vi "CRYNL Interpolation.vi"(10 "y in":dbl[](array[numeric]), 11 "x in":dbl[](array[numeric])) -> (2 "y out":dbl[](array[numeric]))   [LabVIEW 2013]
uses:
  <vilib>/Analysis/4window.llb/Hanning Window (DBL).vi
  <vilib>/Analysis/4window.llb/AllCosWindow (DBL).vi
  <vilib>/Analysis/NI_AALPro.lvlib
panel:
  out "Raw and Interpolated Data":cluster{"x in":dbl[], "y in":dbl[]}[](graph)
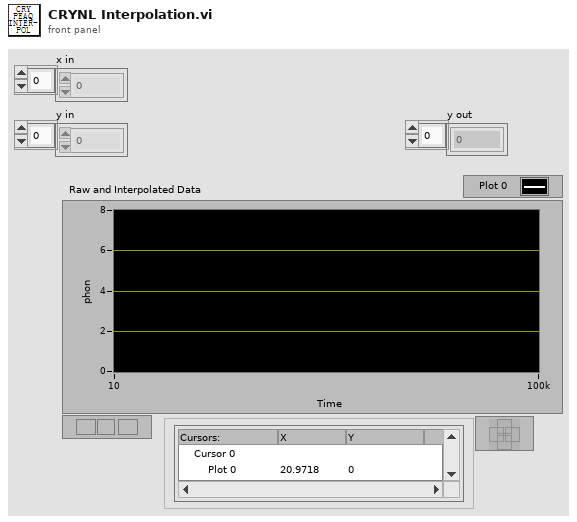
[diagram p1: front panel]
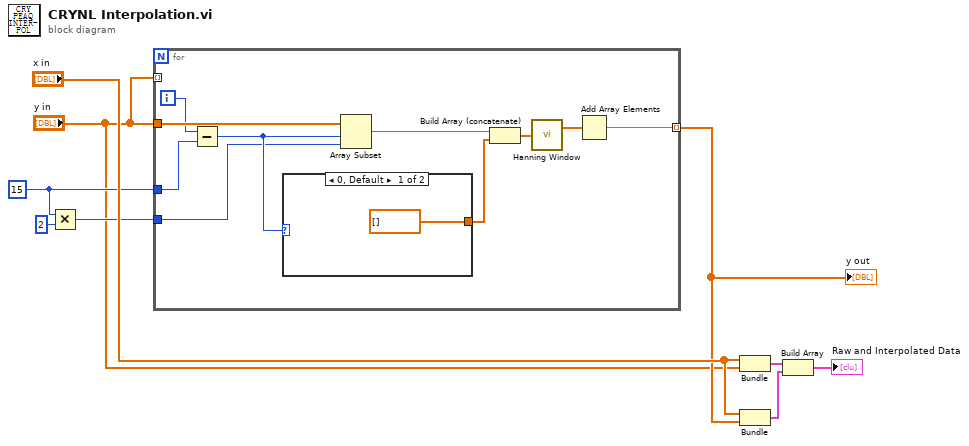
[diagram p0: block diagram]
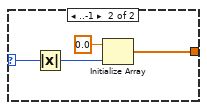
[diagram p2: hidden frame]
diagram:
  w6 = 15 ("y")
  n1 = Multiply(x=w6, y=2) -> (x*y=w4:i32)
  n2 = for {
    tunnel: "y in" -> [w19]
    tunnel: w6 -> [w17]
    tunnel: [w16] -> w3 mode=indexing
    tunnel: w4 -> [w14]
    tunnel: "y in" -> [_] mode=indexing
    i -> [w18]
    n3 = Subtract(x=w18, y=w17) -> (x-y=w15:i32)
    n4 = case shown="0, Default" w15 {
      selector: w15 -> [_ w24]
      tunnel: [dbl[] [] w21] -> w12
      frame 0, Default {
      }
      frame ..-1 {
        n5 = Absolute Value(x=w24) -> (abs(x)=w22:i32)
        n6 = Initialize Array(0.0, w22) -> (w21:dbl[])
      }
    }
    n7 = Array Subset(array=w19, index=w15, length=w14) -> (w13:dbl[])
    n8 = Build Array (concatenate)(w13, w12) -> (w11:dbl[])
    n9 = call-poly <vilib>:"Hanning Window.vi"("X"=w11) -> ("Windowed X"=w10:dbl[])  [unwired: 1 out]
    n10 = Add Array Elements(numeric array=w10) -> (sum=w16:dbl)
  }
  "y out" <- w3
  n11 = Bundle("x in"="x in", "y in"="y in") -> (w8:cluster{"x in":dbl[], "y in":dbl[]})  [unwired: 1 in]
  n12 = Bundle("x in"="x in", w3) -> (w9:cluster{"x in":dbl[], dbl[]})  [unwired: 1 in]
  n13 = Build Array(w8, w9) -> (→"Raw and Interpolated Data":cluster{"x in":dbl[], "y in":dbl[]}[])
